vi "Configure Servo.vi"(0 "Arduino Resource":T1={"VISA resource"="", "Board Type"=enum."Arduino Uno", "Connection Type"=enum."USB / Serial", "Bytes Per Packet (15)"=15}, 5 "Servo Number (0)":u8, 7 "DIO Pin (2)":u8=2, 11 "error in":errorcluster) -> (4 "Arduino Resource":T1={"VISA resource"="", "Board Type"=enum."Arduino Uno", "Connection Type"=enum."USB / Serial", "Bytes Per Packet (15)"=15}, 15 "error out":errorcluster)   [LabVIEW 2011, in "LabVIEW Interface for Arduino.lvlib"]
doc: "Configure Servo assigns a digital output pin to a servo. Before calling Configure Servo you must set the number of servos to use by calling the Set Number of Servos VI."
uses:
  LabVIEW Interface for Arduino.lvlib
  Private/Type Defs/Arduino Resource.ctl
  Private/Type Defs/Board Type.ctl
  Private/Type Defs/Command.ctl
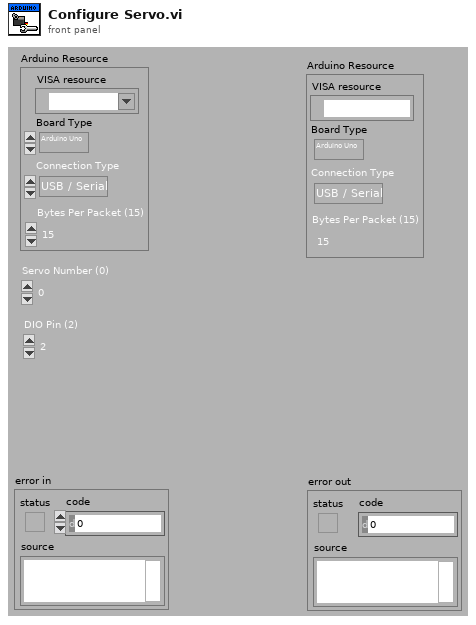
[diagram p1: front panel]
types:
  T1 = typedef "LabVIEW Interface for Arduino.lvlib/Arduino Resource.ctl" = cluster{"VISA resource":refnum<visa-resource-name>, "Board Type":T2, "Connection Type":enum8{"USB / Serial"}, "Bytes Per Packet (15)":u8}
  T2 = typedef "LabVIEW Interface for Arduino.lvlib/Board Type.ctl" = enum16{"Arduino Uno", "Dimuelanove w/Atmega 328", "Mega 2560", "Chipkit Uno32", "Chipkit Max32"}
  T3 = typedef "LabVIEW Interface for Arduino.lvlib/Command.ctl" = enum8{"setArduinoMode", "flushSerial", "setPinMode", "digitalWritePin", "digitalWritePort", "tone", "digitalReadPin", "digitalReadPort", "analogReadPin", "analogReadPort", "pwmWritePin", "pwmWritePort", "sevenSegment_Configure", "sevenSegment_Write", "I2C Init", "I2C Write", "I2C Read", "SPI Init", "SPI Set Bit Order", "SPI Set Clock Divider", "SPI Set Data Mode", "SPI Send / Receive", "SPI Close", "Servo Set Num Servos", "Servo Config Servo", "Servo Write Angle", "Servo Read Angle", "Servo Write Pulse Width", "Servo Read Pulse Width", "Servo Detach", "LCD Init", "LCD Set Size", "LCD Set Cursor Mode", "LCD Clear", "LCD Set Cursor Position", "LCD Print", "LCD Display Power", "LCD Scroll Display", "LCD Autoscroll", "LCD Print Direction", "LCD Create Custom Char", "LCD Print Custom Char", "contAcqOn", "contAcqOff", "getFirmwareVersion", "FiniteSampleStart"}
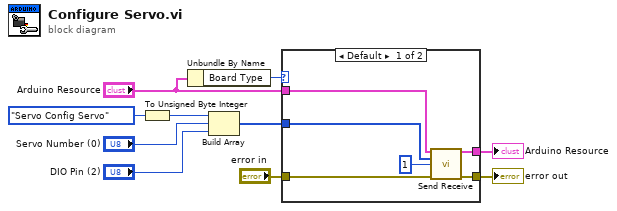
[diagram p0: block diagram]
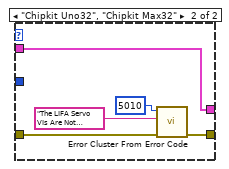
[diagram p2: hidden frame]
diagram:
  n1 = To Unsigned Byte Integer(number=Command."Servo Config Servo" ("Command")) -> (unsigned 8bit integer=w9:u8)
  n2 = Unbundle By Name("Arduino Resource") -> ("Board Type"=w5:T2)
  n3 = Build Array(w9, "Servo Number (0)", "DIO Pin (2)") -> (w1:u8[])
  n4 = case shown="Default" w5 {
    tunnel: "error in" -> [w15 w19]
    tunnel: [w12 w18] -> w2
    tunnel: "Arduino Resource" -> [w14 w17]
    tunnel: [w13 w17] -> w3
    tunnel: w1 -> [w11 _]
    frame Default {
      n5 = call "Send Receive.vi"("Arduino Resource"=w14, "Data"=w11, "Bytes To Read (0)"=u8 1, "error in"=w15) -> ("Arduino Resource"=w13:T1, "error out"=w12:errorcluster)  [unwired: 9 in, 1 out]
    }
    frame "Chipkit Uno32", "Chipkit Max32" {
      n6 = call <vilib>:"Error Cluster From Error Code.vi"("error in (no error)"=w19, "error message (\"\")"="The LIFA Servo VIs Are Not Supported On Chipkit Targets." ("source"), "error code (0)"=5010) -> ("error out"=w18:errorcluster)  [unwired: 6 in]
    }
  }
  "Arduino Resource" <- w3
  "error out" <- w2
